vi "Keithley 6517A LTCC Single Read with Scanner Select.vi"(8 "error in":T1, 9 "Read Displays":bool=TRUE, 10 "Scanner Channel":i16=1 min=1 max=10 step=1, 11 "GPIB address":string="1:27") -> (0 "error out":T1, 1 "time and date stamp":string="03:56:06.00,15-Jul-  94", 2 "Time":string="03:56:06.00", 3 "measurement":dbl=-0.063534 format="%.6e", 4 "secondary display":string="\"               Vsource:+000.000V\"\n", 5 "units":string="VDC", 6 "reading #":dbl=1512.0, 7 "primary display":string="\"-0.063534 V CH01    \"\n")   [LabVIEW 2013]
doc: "This VI takes a single reading from the 6517. The data returned includes the reading, timestamp, units, and reading#."
panel:
  out "Raw Readback":string="-0.063534E+00VDC,03:56:06.00,15-Jul-  94,+01512RDNG#\n"
  # "(A)"
  # "ON\nOFF"
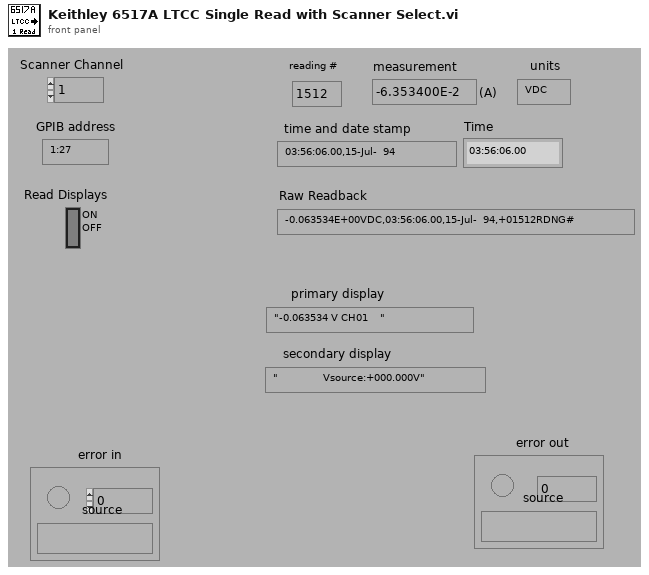
[diagram p1: front panel]
types:
  T1 = cluster{"error":bool, "code":i32, "source":string}
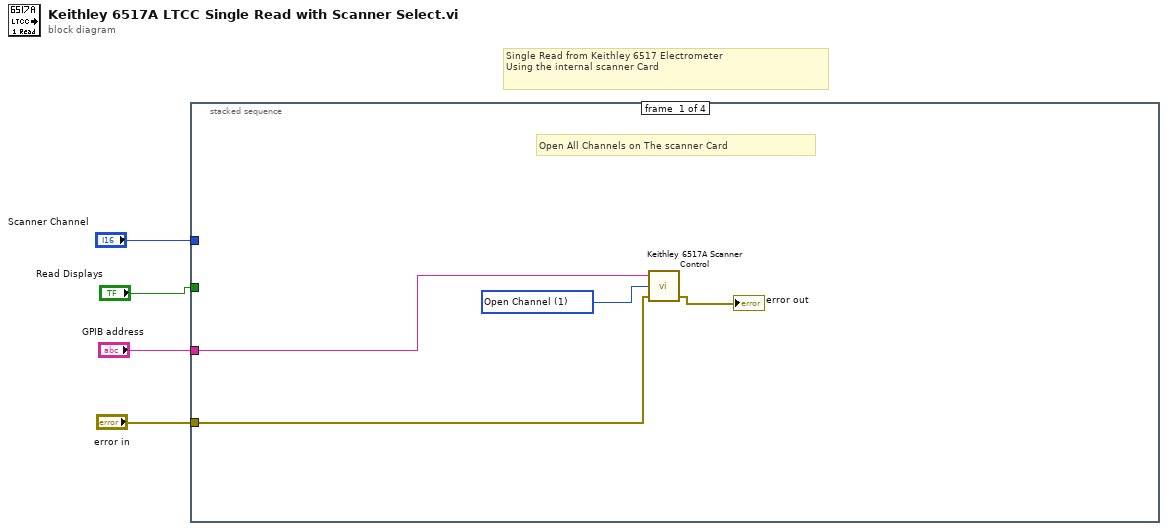
[diagram p0: block diagram]
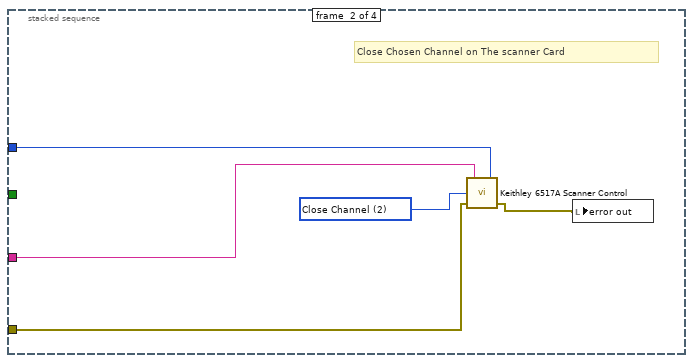
[diagram p2: hidden frame]
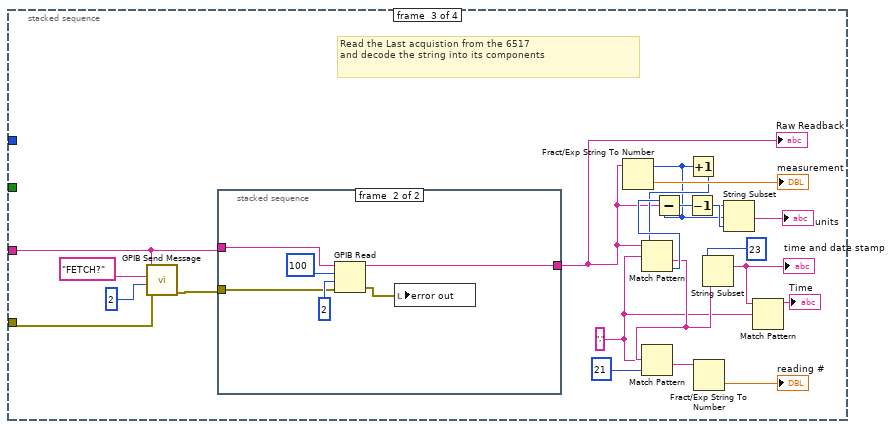
[diagram p3: hidden frame]
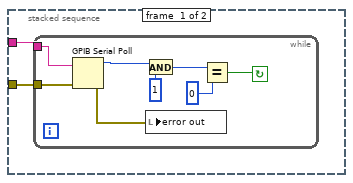
[diagram p4: hidden frame]
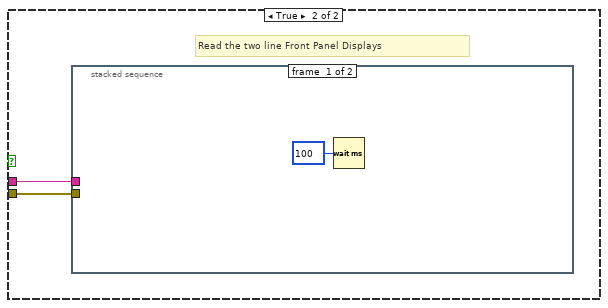
[diagram p6: hidden frame]
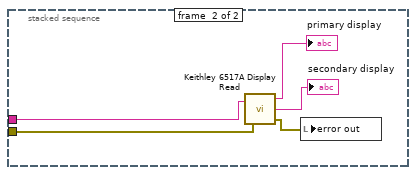
[diagram p7: hidden frame]
diagram:
  # "Single Read from Keithley 6517 Electrometer \nUsing the internal scanner Card"
  n1 = stacked-sequence {
    tunnel: "GPIB address" -> [w5 w11 w19 w52]
    tunnel: "error in" -> [w8 w13 w17 w51]
    tunnel: "Scanner Channel" -> [_ w9 _ _]
    tunnel: "Read Displays" -> [_ _ _ w53]
    frame #0 {
      w7 = u16 1 items=["Open All", "Open Channel", "Close Channel", "Scan List"] ("Scanner Control")
      # "Open All Channels on The scanner Card"
      n2 = call "Keithley 6517A Scanner Control.vi"("error in"=w8, "Scanner Control"=w7, "GPIB address"=w5) -> ("error out"=→"error out":T1)  [unwired: 2 in]
    }
    frame #1 {
      w12 = u16 2 items=["Open All", "Open Channel", "Close Channel", "Scan List"] ("Scanner Control")
      # "Close Chosen Channel on The scanner Card"
      n3 = call "Keithley 6517A Scanner Control.vi"("Open / Close Internal Scanner Channel"=w9, "error in"=w13, "Scanner Control"=w12, "GPIB address"=w11) -> ("error out"=w10:T1)  [unwired: 1 in]
      n4 = local write "error out"(w10) -> ()
    }
    frame #2 {
      w16 = ","
      # "Read the Last acquistion from the 6517\nand decode the string into its components"
      n5 = call "GPIB Send Message.vi"("address string"=w19, "write buffer"="FETCH?", "write mode (set END:0)"=2, "error in"=w17) -> ("error out"=w20:T1)  [unwired: 3 in, 2 out]
      n6 = stacked-sequence {
        tunnel: [_ w50] -> w18
        tunnel: w20 -> [w35 w47]
        tunnel: w19 -> [w36 w46]
        frame #0 {
          n7 = while {
            tunnel: w36 -> [w39]
            tunnel: w35 -> [w38]
            stop <- w43 continue-if-true
            n8 = GPIB Serial Poll(0:w39, 1:w38) -> (2:w42:i16, 4:w37:errorcluster)  [unwired: 1 out]
            n9 = And(x=w42, y=1) -> (x .and. y?=w40:i32)
            n10 = local write "error out"(w37) -> ()
            n11 = Equal?(x=w40, y=0) -> (x = y?=w43:bool)
          }
        }
        frame #1 {
          n12 = GPIB Read(0:w46, 1:100, 2:2, 3:w47) -> (5:w50:string, 7:w45:errorcluster)  [unwired: 1 in, 1 out]
          n13 = local write "error out"(w45) -> ()
        }
      }
      "Raw Readback" <- w18
      n14 = Fract/Exp String To Number(string=w18) -> (offset past number=w23:i32, number=→"measurement":dbl)  [unwired: 3 in]
      n15 = Increment(x=w23) -> (x+1=w24:i32)
      n16 = Match Pattern(string=w18, regular expression=w16, offset (0)=w24) -> (after substring=w26:string, offset past match=w30:i32)  [unwired: 2 out]
      n17 = Match Pattern(string=w26, regular expression=w16, offset (0)=21) -> (after substring=w31:string)  [unwired: 3 out]
      n18 = Subtract(x=w30, y=w23) -> (x-y=w28:i32)
      n19 = Decrement(x=w28) -> (x-1=w29:i32)
      n20 = Fract/Exp String To Number(string=w31) -> (number=→"reading #":dbl)  [unwired: 3 in, 1 out]
      n21 = String Subset(string=w26, length (rest)=23) -> (substring=w15:string)  [unwired: 1 in]
      "time and date stamp" <- w15
      n22 = String Subset(string=w18, offset (0)=w23, length (rest)=w29) -> (substring=→"units":string)
      n23 = Match Pattern(string=w15, regular expression=w16) -> (before substring=→"Time":string)  [unwired: 1 in, 3 out]
    }
    frame #3 {
      n24 = case shown="False" w53 {
        tunnel: w52 -> [_ w55]
        tunnel: w51 -> [_ w54]
        frame False {
        }
        frame True {
          # "Read the two line Front Panel Displays"
          n25 = stacked-sequence {
            tunnel: w55 -> [_ w61]
            tunnel: w54 -> [_ w60]
            frame #0 {
              n26 = Wait (ms)(milliseconds to wait=u32 100) -> ()  [unwired: 1 out]
            }
            frame #1 {
              n27 = call "Keithley 6517A Display Read.vi"("GPIB address"=w61, "error in"=w60) -> ("primary display"=→"primary display":string, "secondary display"=→"secondary display":string, "error out"=w57:T1)
              n28 = local write "error out"(w57) -> ()
            }
          }
        }
      }
    }
  }
